vi "MessageBox.vi"(8 "error in":errorcluster, 11 "Message Box":refnum<vi>) -> (0 "error out":errorcluster, 3 "MessageBox out":refnum<class "MessageBox.lvclass">)   [LabVIEW 2014, in "MessageBox.lvclass"]
uses:
  MessageBox.lvclass
  MessageBox.lvclass/MessageBox.ctl
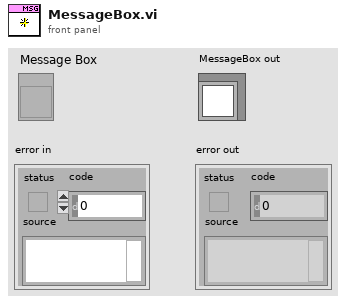
[diagram p1: front panel]
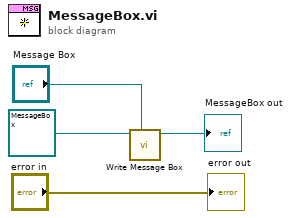
[diagram p0: block diagram]
diagram:
  n1 = call "Write Message Box.vi"("Message Box"="Message Box", "MessageBox in"=refnum<class "MessageBox.lvclass"> refnum) -> ("MessageBox out"=→"MessageBox out":refnum<class "MessageBox.lvclass">)  [unwired: 7 in]
  "error out" <- "error in"
